vi "Write Sub Panel.vi"(8 "error in (no error)":errorcluster, 10 "Sub Panel":refnum<vi>, 11 "subpanel_abstract in":refnum<class "subpanel (abstract).lvclass">) -> (0 "error out":errorcluster, 3 "subpanel_abstract out":refnum<class "subpanel (abstract).lvclass">)   [LabVIEW 2023, in "GUI.lvlib" / "subpanel (abstract).lvclass"]
uses:
  subpanel (abstract).lvclass
  subpanel (abstract).lvclass/subpanel (abstract).ctl
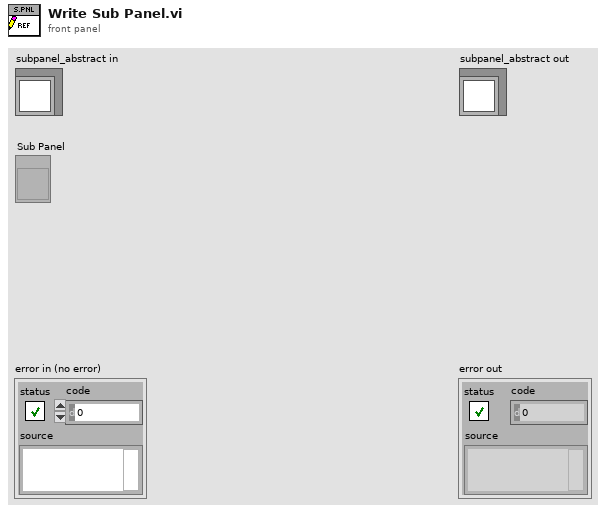
[diagram p1: front panel]
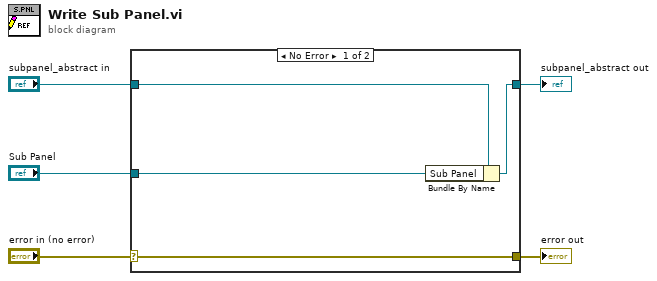
[diagram p0: block diagram]
diagram:
  n1 = case shown="No Error" "error in (no error)" {
    selector: "error in (no error)" -> [w9 w10]
    tunnel: [w9 w10] -> w4
    tunnel: [w7 w11] -> w2
    tunnel: "subpanel_abstract in" -> [w8 w11]
    tunnel: "Sub Panel" -> [w6 _]
    frame No Error {
      n2 = Bundle By Name(cluster=w8, "Sub Panel"=w6) -> (w7:refnum<class "subpanel (abstract).lvclass">)
    }
    frame Error {
    }
  }
  "error out" <- w4
  "subpanel_abstract out" <- w2
